vi "interp_2d_round_up.vi"(10 "z":dbl[](array[numeric]), 11 "prelookup":cluster{"frac":dbl, "num":u8}) -> (3 "z":dbl)   [LabVIEW 2013]
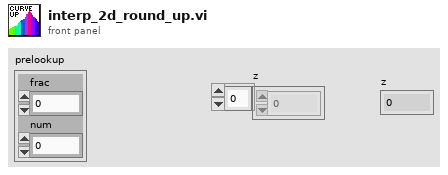
[diagram p1: front panel]
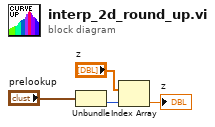
[diagram p0: block diagram]
diagram:
  n1 = Unbundle("prelookup") -> ("num"=w2:u8)  [unwired: 1 out]
  n2 = Index Array(array="z", index=w2) -> (element=→"z":dbl)
